vi "Load Device Channels.vi"(8 "Error In":errorcluster, 11 "LINX Resource":T1) -> (0 "Error Out":errorcluster, 3 "LINX Resource":T1)   [LabVIEW 2020, in "LMH-LINX.lvlib" / "Local IO.lvlib"]
uses:
  Local IO.lvlib
  Type Defs/LINX Ref.ctl
  Type Defs/Platform.ctl
  Type Defs/Interface.ctl
  Device/Type Defs/LINX Device Config.ctl
  Device/Type Defs/TCP Config.ctl
  Device/Type Defs/Channels.ctl
  Utilties/Generate Error.vi
  LMH-LINX.lvlib
  Device/Device.lvlib
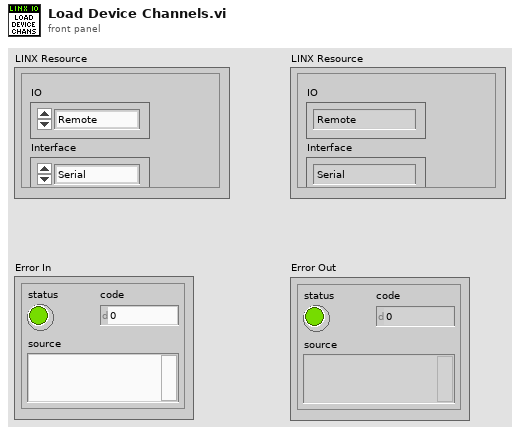
[diagram p1: front panel]
types:
  T1 = typedef "LMH-LINX.lvlib/LINX Ref.ctl" = cluster{"IO":T2, "Interface":T3, "LINX Device Config":T4}
  T2 = typedef "LMH-LINX.lvlib/Platform.ctl" = enum16{"Remote", "Local"}
  T3 = typedef "LMH-LINX.lvlib/Interface.ctl" = enum16{"Serial", "TCP"}
  T4 = typedef "Device.lvlib/LINX Device Config.ctl" = cluster{"Interface":T3, "COM Port":refnum<visa-resource-name>, "TCP Configuration":T5, "Device Family":u8, "Device ID":u8, "Device Name":string, "TCP Ref":refnum<k5>, "Channels":T6}
  T5 = typedef "Device.lvlib/TCP Config.ctl" = cluster{"IP Address":string, "Port":u16}
  T6 = typedef "LMH-LINX.lvlib/Channels.ctl" = cluster{"DI":u8[], "DO":u8[], "AI":u8[], "AO":u8[], "PWM":u8[], "QE":u8[], "UART":u8[], "I2C 2":u8[], "SPI":u8[], "CAN":u8[], "Servo":u8[], "AI Ref (V)":dbl, "AI Resolution (Bits)":u8, "AO Ref (V)":dbl, "AO Resolution (Bits)":u8}
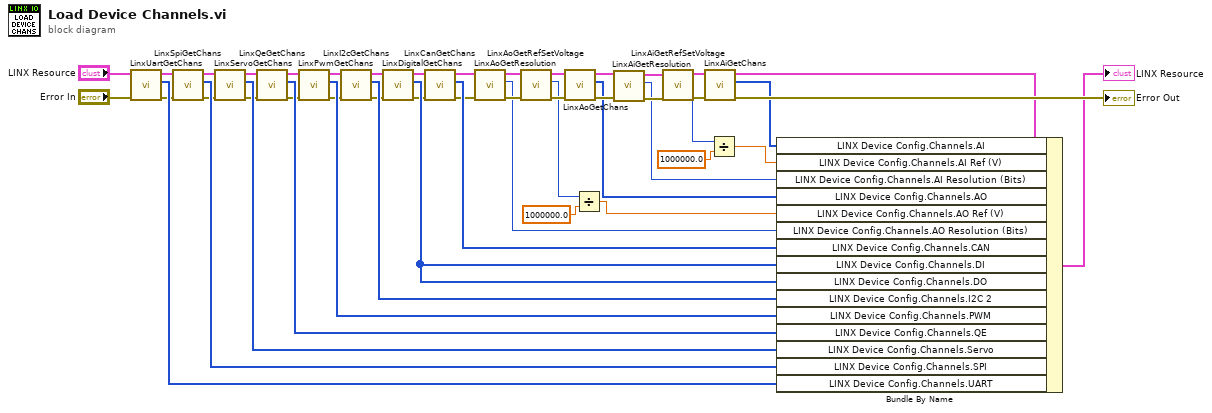
[diagram p0: block diagram]
diagram:
  n1 = call "LinxUartGetChans.vi"("Error In"="Error In", "LINX Resource"="LINX Resource") -> ("Error Out"=w37:errorcluster, "Uart Channels"=w40:u8[], "LINX Resource"=w22:T1)  [unwired: 6 in, 1 out]
  n2 = call "LinxSpiGetChans.vi"("Error In"=w37, "LINX Resource"=w22) -> ("Error Out"=w36:errorcluster, "SPI Channels"=w41:u8[], "LINX Resource"=w23:T1)  [unwired: 6 in, 1 out]
  n3 = call "LinxServoGetChans.vi"("Error In"=w36, "LINX Resource"=w23) -> ("Error Out"=w35:errorcluster, "Servo Channels"=w42:u8[], "LINX Resource"=w24:T1)  [unwired: 6 in, 1 out]
  n4 = call "LinxQeGetChans.vi"("Error In"=w35, "LINX Resource"=w24) -> ("Error Out"=w34:errorcluster, "QE Channels"=w43:u8[], "LINX Resource"=w25:T1)  [unwired: 6 in, 1 out]
  n5 = call "LinxPwmGetChans.vi"("Error In"=w34, "LINX Resource"=w25) -> ("Error Out"=w33:errorcluster, "PWM Channels"=w44:u8[], "LINX Resource"=w26:T1)  [unwired: 6 in, 1 out]
  n6 = call "LinxI2cGetChans.vi"("Error In"=w33, "LINX Resource"=w26) -> ("Error Out"=w32:errorcluster, "I2C Channels"=w45:u8[], "LINX Resource"=w27:T1)  [unwired: 6 in, 1 out]
  n7 = call "LinxDigitalGetChans.vi"("Error In"=w32, "LINX Resource"=w27) -> ("Error Out"=w31:errorcluster, "Digital Channels"=w46:u8[], "LINX Resource"=w28:T1)  [unwired: 6 in, 1 out]
  n8 = call "LinxCanGetChans.vi"("Error In"=w31, "LINX Resource"=w28) -> ("Error Out"=w3:errorcluster, "CAN Channels"=w47:u8[], "LINX Resource"=w2:T1)  [unwired: 6 in, 1 out]
  n9 = call "LinxAoGetResolution.vi"("Error In"=w3, "LINX Resource"=w2) -> ("Error Out"=w4:errorcluster, "AO Resolution"=w1:u8, "LINX Resource"=w5:T1)  [unwired: 7 in]
  n10 = call "LinxAoGetRefSetVoltage.vi"("Error In"=w4, "LINX Resource"=w5) -> ("Error Out"=w18:errorcluster, "AoRef Set"=w15:i32, "LINX Resource"=w17:T1)  [unwired: 7 in]
  n11 = call "LinxAoGetChans.vi"("Error In"=w18, "LINX Resource"=w17) -> ("Error Out"=w11:errorcluster, "AO Channels"=w7:u8[], "LINX Resource"=w12:T1)  [unwired: 6 in, 1 out]
  n12 = Divide(x=w15, y=1000000.0) -> (x/y=w6:dbl)
  n13 = call "LinxAiGetResolution.vi"("Error In"=w11, "LINX Resource"=w12) -> ("Error Out"=w10:errorcluster, "AI Resolution"=w8:u8, "LINX Resource"=w9:T1)  [unwired: 7 in]
  n14 = call "LinxAiGetRefSetVoltage.vi"("Error In"=w10, "LINX Resource"=w9) -> ("Error Out"=w30:errorcluster, "AiRef Set"=w49:u32, "LINX Resource"=w29:T1)  [unwired: 7 in]
  n15 = call "LinxAiGetChans.vi"("Error In"=w30, "LINX Resource"=w29) -> ("Error Out"=→"Error Out":errorcluster, "AI Channels"=w14:u8[], "LINX Resource"=w20:T1)  [unwired: 6 in, 1 out]
  n16 = Divide(x=w49, y=1000000.0) -> (x/y=w13:dbl)
  n17 = Bundle By Name(cluster=w20, "LINX Device Config.Channels.AI"=w14, "LINX Device Config.Channels.AI Ref (V)"=w13, "LINX Device Config.Channels.AI Resolution (Bits)"=w8, "LINX Device Config.Channels.AO"=w7, "LINX Device Config.Channels.AO Ref (V)"=w6, "LINX Device Config.Channels.AO Resolution (Bits)"=w1, "LINX Device Config.Channels.CAN"=w47, "LINX Device Config.Channels.DI"=w46, "LINX Device Config.Channels.DO"=w46, "LINX Device Config.Channels.I2C 2"=w45, "LINX Device Config.Channels.PWM"=w44, "LINX Device Config.Channels.QE"=w43, "LINX Device Config.Channels.Servo"=w42, "LINX Device Config.Channels.SPI"=w41, "LINX Device Config.Channels.UART"=w40) -> (→"LINX Resource":T1)
